vi "Process Phasor Configuration.vi"(7 "PMU Name":string, 11 "Phasor Configuration In":T2) -> (1 "Phasor Types":u8[](array[numeric]), 2 "Phasor Channel Names":string[](array[string]), 3 "Phasor Configuration Out":T1(array[cluster]))   [LabVIEW 2013, in "PMU Recorder Light.lvlib" / "Phasor Data Concentrator.lvclass"]
uses:
  Phasor Data Concentrator.lvclass
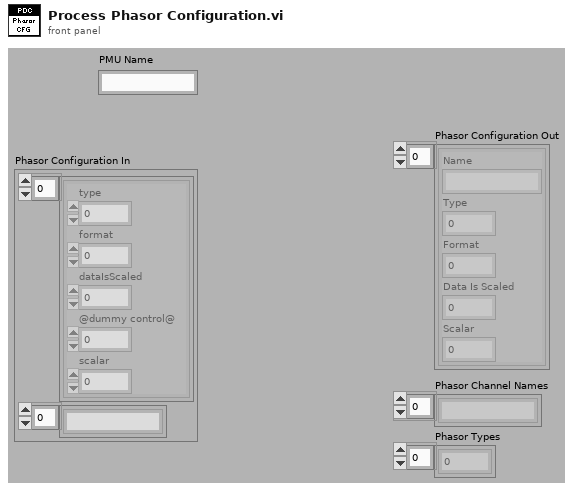
[diagram p1: front panel]
types:
  T1 = cluster{"Name":string, "Type":u8, "Format":u8, "Data Is Scaled":u8, "Scalar":sgl}[]
  T2 = cluster{cluster{"type":u8, "format":u8, "dataIsScaled":u8, "@dummy control@":i8, "scalar":sgl}[], string[]}
  T3 = cluster{"type":u8, "format":u8, "dataIsScaled":u8, "@dummy control@":i8, "scalar":sgl}[]
  T4 = cluster{"Name":string, "Type":u8, "Format":u8, "Data Is Scaled":u8, "Scalar":sgl}
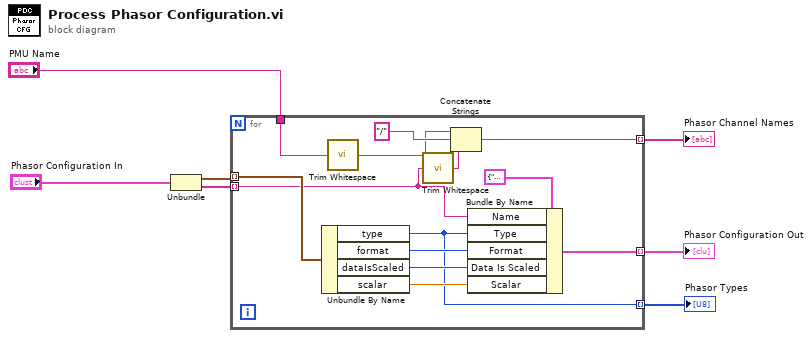
[diagram p0: block diagram]
diagram:
  n1 = Unbundle("Phasor Configuration In") -> (w3:T3, w4:string[])
  n2 = for {
    tunnel: [w19] -> w7 mode=indexing
    tunnel: "PMU Name" -> [w17]
    tunnel: w4 -> [w8] mode=indexing
    tunnel: w3 -> [w15] mode=indexing
    tunnel: [w11] -> w2 mode=indexing
    tunnel: [w10] -> w1 mode=indexing
    n3 = Unbundle By Name(w15) -> ("type"=w10:u8, "format"=w14:u8, "dataIsScaled"=w13:u8, "scalar"=w12:sgl)
    n4 = call <vilib>:"Trim Whitespace.vi"("string"=w17) -> ("trimmed string"=w18:string)  [unwired: 1 in]
    n5 = call <vilib>:"Trim Whitespace.vi"("string"=w8) -> ("trimmed string"=w9:string)  [unwired: 1 in]
    n6 = Concatenate Strings(w18, "/" ("string"), w9) -> (w19:string)
    n7 = Bundle By Name(cluster=T4 {"Name"="", "Type"=0, "Format"=0, "Data Is Scaled"=0, "Scalar"=0.0} ("Phasor Configuration"), "Name"=w8, "Type"=w10, "Format"=w14, "Data Is Scaled"=w13, "Scalar"=w12) -> (w11:T4)
  }
  "Phasor Channel Names" <- w7
  "Phasor Configuration Out" <- w2
  "Phasor Types" <- w1
